vi "Screen_LogFileView.vi"() -> ()   [LabVIEW 2010]
uses:
  030 - EVENTS/EnumFgvEventCommand.ctl
  LogFileViewerAppContext.ctl
  100_PROCESS/01_MessageHandlerProcess/SubVis/LogFileData.ctl
  030 - EVENTS/03 - ToMessageHandlerProcess/ToMessageHandlerEvent.ctl
  030 - EVENTS/03 - ToMessageHandlerProcess/enumMessageCriticity.ctl
  090 - ERRORS/Ctrls/enumLogAndView.ctl
  enumScreen.ctl
  020 - HMI/SubVis/enumDeferPanelUpdate.ctl
panel:
  in  "Liste fichiers LOG":u16(ring) items=["fdfdfdfd"]
  in  "Messages viewer":i32(listbox)
  in  "Bouton menu principal":bool
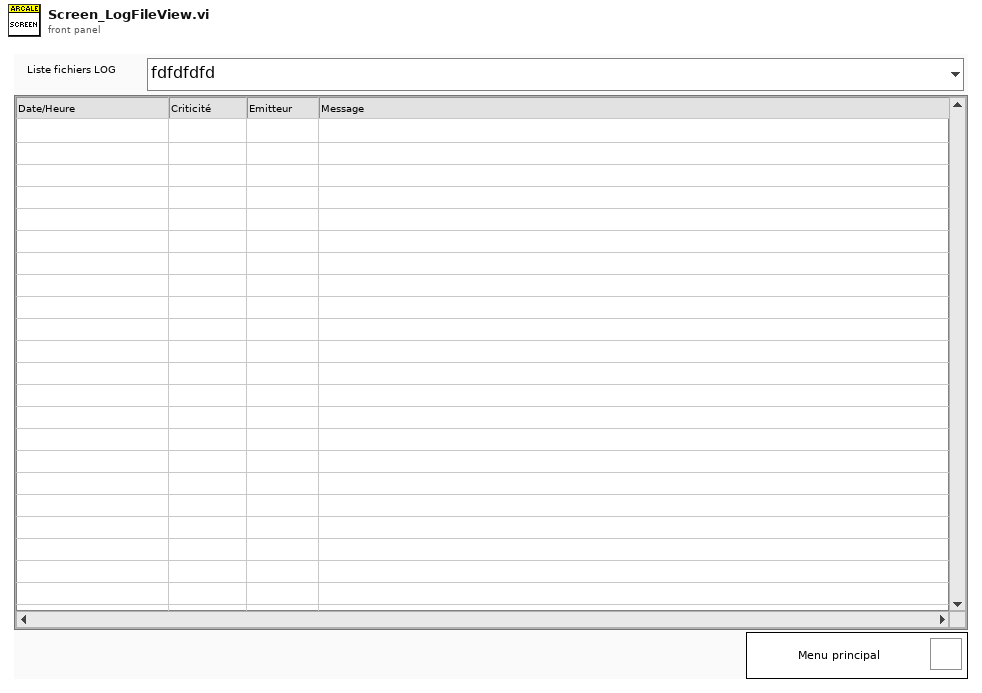
[diagram p1: front panel]
types:
  T1 = typedef "enumLogAndView.ctl" = enum16{"Log only", "Log and view"}
  T2 = typedef "LogFileViewerAppContext.ctl" = cluster{"LogFilePathArray":path[], "Current LogFile Messages":T3}
  T3 = typedef "LogFileData.ctl" = cluster{"MessageArray":T4[]}
  T4 = typedef "ToMessageHandlerEvent.ctl" = cluster{"date / time":timestamp, "Criticity":T5, "Emitter":string, "Message":string}
  T5 = typedef "enumMessageCriticity.ctl" = enum16{"No error", "Info", "Warning", "Error", "Fatal error"}
  T6 = typedef "EnumFgvEventCommand.ctl" = enum16{"Setup", "Cleanup", "Get"}
  T7 = typedef "enumScreen.ctl" = enum16{"Test screen", "Ecran principal", "LOG", "Setup", "Popup : About", "Popup : View last message", "Popup : WebBrowser help", "Traduction"}
  T8 = typedef "enumDeferPanelUpdate.ctl" = enum16{"suspend layout", "resume layout"}
  T9 = typedef "ToScreensCommand.ctl" = enum16{"Stop screen", "Stop all screens"}
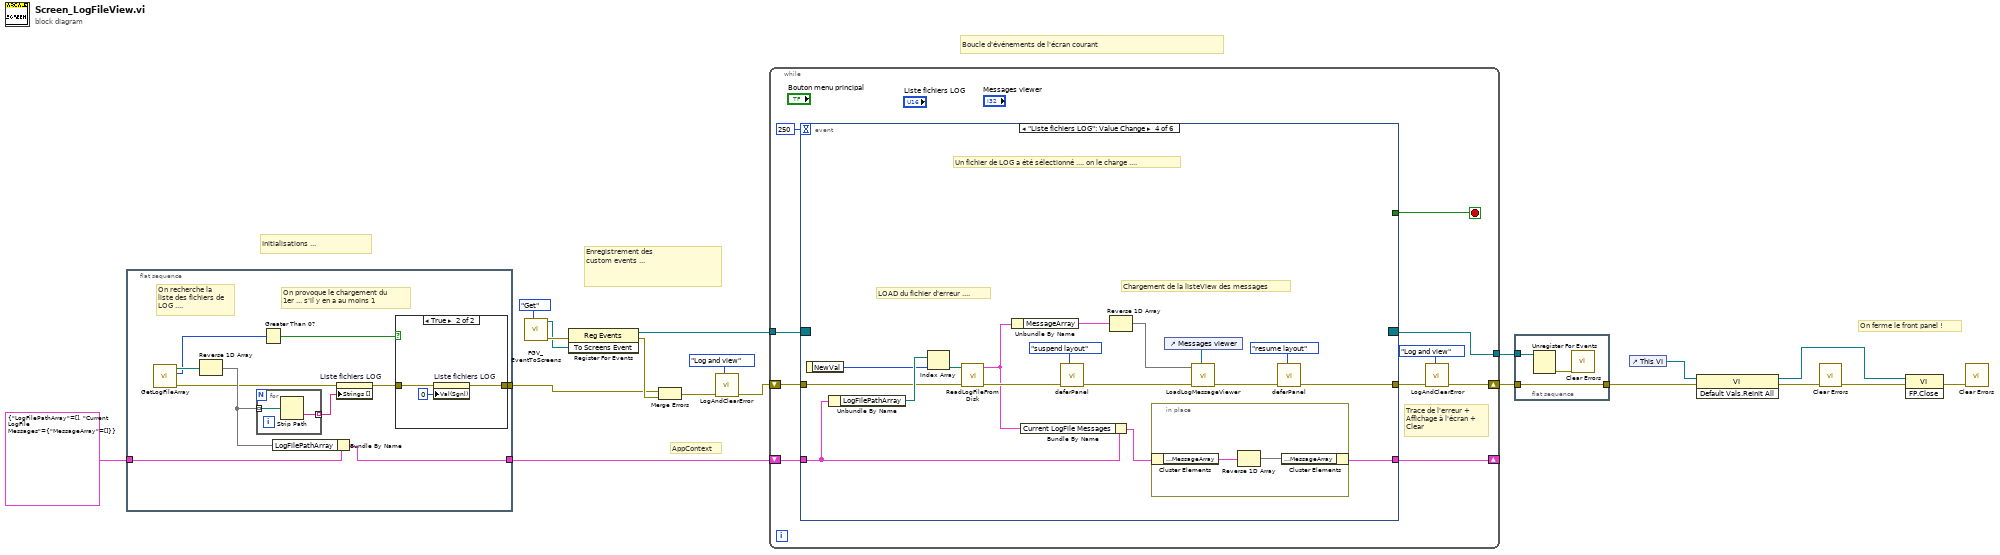
[diagram p0: block diagram]
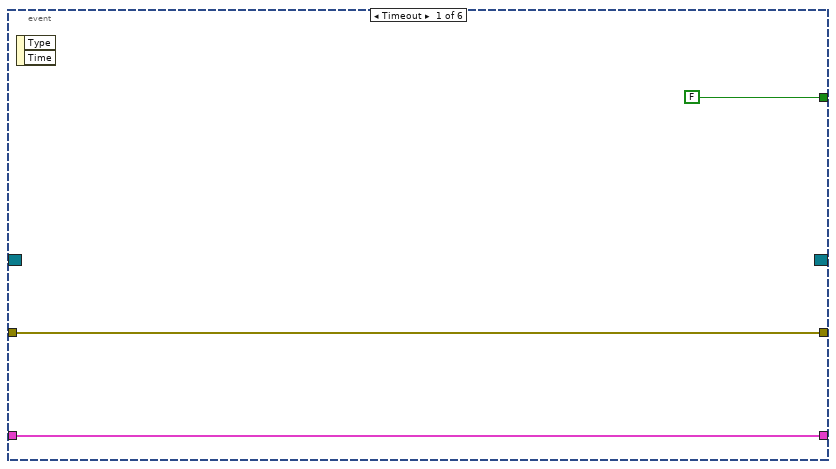
[diagram p3: hidden frame]
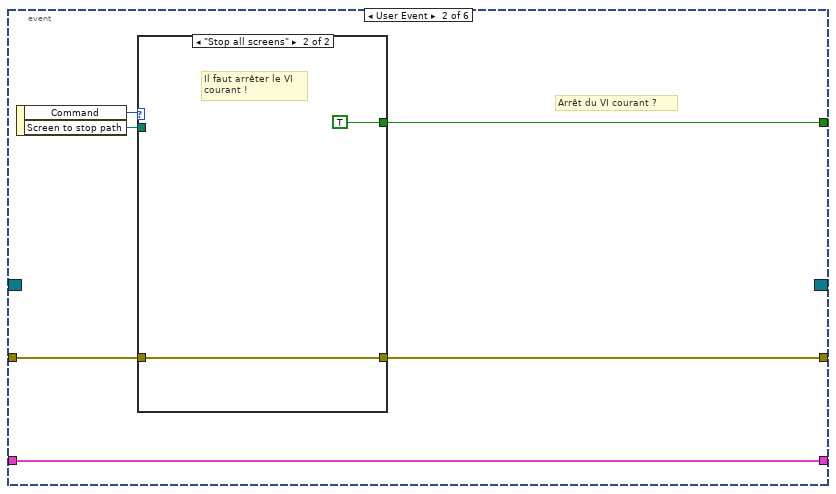
[diagram p4: hidden frame]
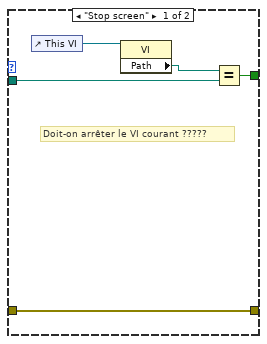
[diagram p5: hidden frame]
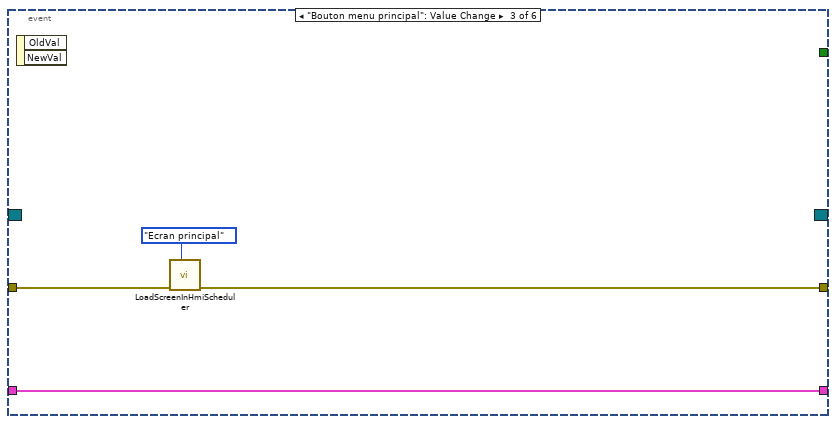
[diagram p6: hidden frame]
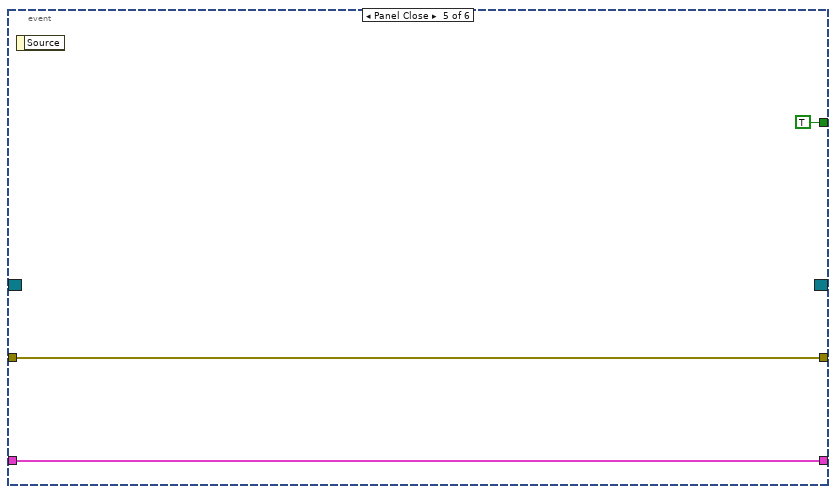
[diagram p7: hidden frame]
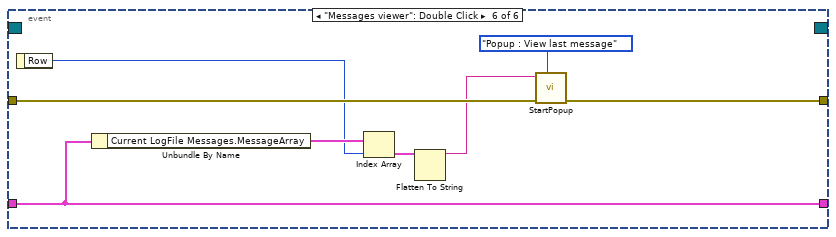
[diagram p8: hidden frame]
diagram:
  # "AppContext"
  # "Enregistrement des\ncustom events ..."
  # "Initialisations ..."
  # "On ferme le front panel !"
  # "Boucle d'événements de l'écran courant"
  n1 = flat-sequence {
    tunnel: T2 {"LogFilePathArray"=[], "Current LogFile Messages"={"MessageArray"=[]}} ("AppConfig") -> [w28]
    tunnel: [w27] -> w10
    tunnel: [w21] -> w9
    frame #0 {
      # "On provoque le chargement du\n1er ... s'il y en a au moins 1"
      # "On recherche la\nliste des fichiers de\nLOG ...."
      n2 = call "GetLogFileArray.vi"() -> ("error out"=w25:errorcluster, "LogFileNumber"=w24:u32, "LogFileArray"=w29:path[])  [unwired: 9 in]
      n3 = Reverse 1D Array(array=w29) -> (reversed array=w26:path[])
      n4 = for {
        tunnel: w26 -> [w35] mode=indexing
        tunnel: [w34] -> w23 mode=indexing
        n5 = Strip Path(path=w35) -> (name=w34:string)  [unwired: 1 out]
      }
      n6 = Greater Than 0?(x=w24) -> (x > 0?=w20:bool)
      n7 = Bundle By Name(cluster=w28, "LogFilePathArray"=w26) -> (w27:T2)
      n8 = property on="Liste fichiers LOG" class="Ring (strict)"(error in=w25, "Strings []"=w23) -> (error out=w22:errorcluster)  [unwired: 1 in, 1 out]
      n9 = case shown="True" w20 {
        tunnel: w22 -> [w30 w33]
        tunnel: [w30 w32] -> w21
        frame False {
        }
        frame True {
          n10 = property on="Liste fichiers LOG" class="Ring (strict)"(error in=w33, "Val(Sgnl)"=u16 0 ("Value (Signaling)")) -> (error out=w32:errorcluster)  [unwired: 1 in, 1 out]
        }
      }
    }
  }
  n11 = call "FGV_EventToScreens.vi"("Command"=EnumFgvEventCommand."Get") -> ("error out"=w19:errorcluster, "To Screens Event"=w18:refnum<user-event>)  [unwired: 9 in]
  n12 = register-events(error in=w19, w18) -> (reference out=w17:refnum<event-registration>, error out=w12:errorcluster)  [unwired: 1 in]
  n13 = Merge Errors(w9, w12) -> (w7:errorcluster)
  n14 = call "LogAndClearError.vi"("Log and view ?"=enumLogAndView."Log and view", "error in (no error)"=w7) -> ("error out"=w6:errorcluster)  [unwired: 9 in]
  n15 = while {
    tunnel: w17 -> [w45]
    shift-right: [w39] -> w15
    shift-left: w6 -> [w44]
    tunnel: [w43] -> w16
    shift-right: [w40] -> _
    shift-left: w10 -> [w41]
    stop <- w42 stop-if-true
    # "Trace de l'erreur +\nAffichage à l'écran +\nClear"
    n16 = event shown="[3] \"Liste fichiers LOG\": Value Change" {
      selector: w45 -> [_ _ _ _ _ _]
      dyn-events: [_ _ _ _ _ _] -> w43
      timeout: 250 -> [_ _ _ _ _ _]
      tunnel: w44 -> [w48 w53 w65 w80 w86 w94]
      tunnel: [w48 w52 w63 w71 w86 w88] -> w38
      tunnel: [FALSE w50 _ _ TRUE _] -> w42
      tunnel: w41 -> [w46 w49 w62 w82 w85 w89]
      tunnel: [w46 w49 w62 w66 w85 w89] -> w40
      event Timeout {
        n17 = event-data() -> ()  [unwired: 1 in, 2 out]
      }
      event User Event {
        # "Arrêt du VI courant ?"
        n18 = event-data() -> ("Command"=w54:T9, "Screen to stop path"=w51:path)  [unwired: 1 in]
        n19 = case shown="\"Stop all screens\"" w54 {
          tunnel: w53 -> [w59 w60]
          tunnel: [w59 w60] -> w52
          tunnel: w51 -> [w56 _]
          tunnel: [w55 TRUE] -> w50
          frame "Stop screen" {
            # "Doit-on arrêter le VI courant ?????"
            n20 = control-ref of="This VI"() -> (w58:refnum<vi>)
            n21 = property class="VI"(reference=w58) -> ("Path"=w57:path)  [unwired: 1 in, 2 out]
            n22 = Equal?(x=w57, y=w56) -> (x = y?=w55:bool)
          }
          frame "Stop all screens" {
            # "Il faut arrêter le VI\ncourant !"
          }
        }
      }
      event "Bouton menu principal": Value Change {
        n23 = event-data() -> ()  [unwired: 1 in, 2 out]
        n24 = call "LoadScreenInHmiScheduler.vi"("Enum Screen"=enumScreen."Ecran principal", "error in (no error)"=w65) -> ("error out"=w63:errorcluster)  [unwired: 9 in]
      }
      event "Liste fichiers LOG": Value Change {
        # "Chargement de la listeView des messages"
        # "LOAD du fichier d'erreur ...."
        # "Un fichier de LOG a été sélectionné .... on le charge ...."
        n25 = event-data() -> ("NewVal"=w79:u16)  [unwired: 1 in]
        n26 = Unbundle By Name(w82) -> ("LogFilePathArray"=w81:path[])
        n27 = Index Array(array=w81, index=w79) -> (element=w78:path)
        n28 = call "ReadLogFileFromDisk.vi"("error in (no error)"=w80, "Log File path"=w78) -> ("error out"=w76:errorcluster, "Messages"=w70:T3)  [unwired: 8 in]
        n29 = Unbundle By Name(w70) -> ("MessageArray"=w69:T4[])
        n30 = Bundle By Name(cluster=w82, "Current LogFile Messages"=w70) -> (w67:T2)
        n31 = call "deferPanel.vi"("EnumDeferPanel"=enumDeferPanelUpdate."suspend layout", "errorIn"=w76) -> ("error out"=w75:errorcluster)  [unwired: 9 in]
        n32 = Reverse 1D Array(array=w69) -> (reversed array=w68:T4[])
        n33 = in-place {
          n34 = in-place-cluster #1(w67) -> ("Current LogFile Messages.MessageArray"=w84:T4[])
          n35 = Reverse 1D Array(array=w84) -> (reversed array=w83:T4[])
          n36 = in-place-cluster #1("Current LogFile Messages.MessageArray"=w83) -> (w66:T2)
        }
        n37 = control-ref of="Messages viewer"() -> (w77:refnum<vi>)
        n38 = call "LoadLogMessageViewer.vi"("Messages viewer"=w77, "error In"=w75, "MessageArray"=w68) -> ("error out"=w72:errorcluster)  [unwired: 8 in]
        n39 = call "deferPanel.vi"("EnumDeferPanel"=enumDeferPanelUpdate."resume layout", "errorIn"=w72) -> ("error out"=w71:errorcluster)  [unwired: 9 in]
      }
      event Panel Close {
        n40 = event-data() -> ()  [unwired: 1 in, 1 out]
      }
      event "Messages viewer": Double Click {
        n41 = event-data() -> ("Row"=w92:i32)  [unwired: 1 in]
        n42 = Unbundle By Name(w89) -> ("Current LogFile Messages.MessageArray"=w93:T4[])
        n43 = Index Array(array=w93, index=w92) -> (element=w91:T4)
        n44 = Flatten To String(anything=w91) -> (data string=w90:string)  [unwired: 3 in, 2 out]
        n45 = call "StartPopup.vi"("Popup"=enumScreen."Popup : View last message", "error in (no error)"=w94, "String parameter"=w90) -> ("error out"=w88:errorcluster)  [unwired: 8 in]
      }
    }
    n46 = call "LogAndClearError.vi"("Log and view ?"=enumLogAndView."Log and view", "error in (no error)"=w38) -> ("error out"=w39:errorcluster)  [unwired: 9 in]
  }
  n47 = flat-sequence {
    tunnel: w16 -> [w98]
    tunnel: w15 -> [w96]
    tunnel: [w96] -> w4
    frame #0 {
      n48 = Unregister For Events(event registration refnum=w98) -> (error out=w97:errorcluster)  [unwired: 1 in]
      n49 = call <vilib>:"Clear Errors.vi"("error in (no error)"=w97) -> ()  [unwired: 6 in, 1 out]
    }
  }
  n50 = control-ref of="This VI"() -> (w3:refnum<vi>)
  n51 = invoke class="VI" method="Default Vals.Reinit All"(reference=w3, error in=w4) -> (reference out=w2:refnum<vi>, error out=w5:errorcluster)  [unwired: 1 in, 1 out]
  n52 = call <vilib>:"Clear Errors.vi"("error in (no error)"=w5) -> ("error out"=w1:errorcluster)  [unwired: 6 in]
  n53 = invoke class="VI" method="FP.Close"(reference=w2, error in=w1) -> (error out=w14:errorcluster)  [unwired: 1 in, 2 out]
  n54 = call <vilib>:"Clear Errors.vi"("error in (no error)"=w14) -> ()  [unwired: 6 in, 1 out]
